vi "Ethernet Config Stress Test.vi"() -> ()   [LabVIEW 2021]
uses:
  Ethernet/Ethernet.lvclass
  Ethernet/Config Types/Ethernet Settings.ctl
panel:
  in  "stop":bool
  out "Iteration":i32
  out "UDP Read good?":bool
  out "TCP Read good?":bool
  out "UDP W/R?":bool
  out "TCP W/R?":bool
  out "error out":errorcluster
  out "Configuration Error?":bool
  out "Settings equal?":bool
  out "Ethernet Settings":T1
  in  "UDP port":u16=54321
  in  "TCP port":u16=12345
  in  "Box IP address":string="192.168.1.100"
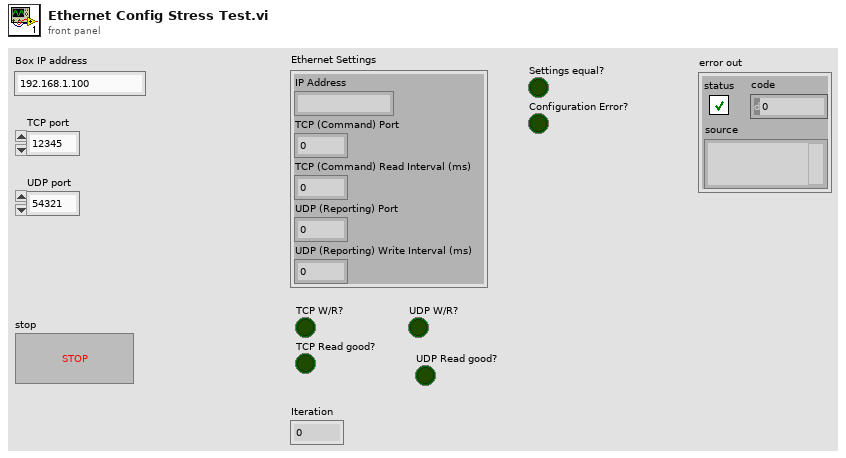
[diagram p1: front panel]
types:
  T1 = typedef "Battery Simulator 1200 LabVIEW Driver.lvlib/Ethernet.lvclass/Ethernet Settings.ctl" = cluster{"IP Address":string, "TCP (Command) Port":u16, "TCP (Command) Read Interval (ms)":u32, "UDP (Reporting) Port":u16, "UDP (Reporting) Write Interval (ms)":u32}
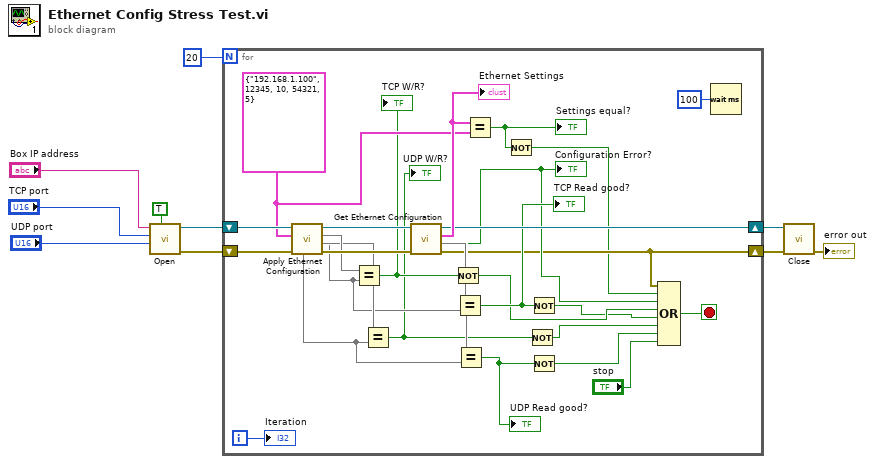
[diagram p0: block diagram]
diagram:
  n1 = call "Open.vi"("Connect for Config Only? (F)"=TRUE, "UDP port"="UDP port", "TCP port"="TCP port", "Box IP address"="Box IP address") -> ("error out"=w10:errorcluster, "ENET out"=w9:refnum<class "Ethernet.lvclass">)  [unwired: 6 in]
  n2 = for {
    N: 20 -> [_]
    shift-right: [w19] -> w3
    shift-left: w10 -> [w39]
    shift-right: [w33] -> w2
    shift-left: w9 -> [w38]
    i -> [w21]
    stop <- w12 stop-if-true
    w34 = T1 {"IP Address"="192.168.1.100", "TCP (Command) Port"=12345, "TCP (Command) Read Interval (ms)"=10, "UDP (Reporting) Port"=54321, "UDP (Reporting) Write Interval (ms)"=5} ("Ethernet Settings")
    n3 = call "Apply Ethernet Configuration.vi"("error in (no error)"=w39, "Ethernet Settings"=w34, "Ethernet in"=w38) -> ("error out"=w37:errorcluster, 1:w29, 2:w32, "Ethernet out"=w36:refnum<class "Ethernet.lvclass">, 4:w31, 6:w27)  [unwired: 3 in]
    n4 = Equal?(x=w32, y=w29) -> (x = y?=w25:bool)
    "TCP W/R?" <- w25
    n5 = Equal?(x=w31, y=w27) -> (x = y?=w23:bool)
    "UDP W/R?" <- w23
    n6 = call "Get Ethernet Configuration.vi"("error in (no error)"=w37, "Ethernet in"=w36) -> ("error out"=w19:errorcluster, "Configuration Error?"=w20:bool, "Ethernet Settings"=w35:T1, "Ethernet out"=w33:refnum<class "Ethernet.lvclass">, 4:w30, 6:w28)  [unwired: 4 in]
    "Ethernet Settings" <- w35
    "Configuration Error?" <- w20
    n7 = Not(x=w25) -> (.not. x?=w17:bool)
    n8 = Equal?(x=w30, y=w29) -> (x = y?=w24:bool)
    "TCP Read good?" <- w24
    n9 = Equal?(x=w28, y=w27) -> (x = y?=w22:bool)
    "UDP Read good?" <- w22
    n10 = Equal?(x=w35, y=w34) -> (x = y?=w26:bool)
    "Settings equal?" <- w26
    n11 = Not(x=w26) -> (.not. x?=w18:bool)
    n12 = Not(x=w23) -> (.not. x?=w15:bool)
    n13 = Not(x=w24) -> (.not. x?=w16:bool)
    n14 = Not(x=w22) -> (.not. x?=w14:bool)
    n15 = Compound Arithmetic op=OR(w19, w18, w20, w17, w16, w15, w14, "stop") -> (w12:bool)
    n16 = Wait (ms)(milliseconds to wait=u32 100) -> ()  [unwired: 1 out]
    "Iteration" <- w21
  }
  n17 = call-dynamic "Close.vi"("error in (no error)"=w3, "ENET in"=w2) -> ("error out"=→"error out":errorcluster)  [unwired: 9 in]
